vi "Flip FLop D (2).vi"() -> ()   [LabVIEW 2018]
panel:
  out "Q0*":bool
  in  "D0":bool
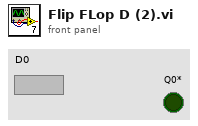
[diagram p1: front panel]
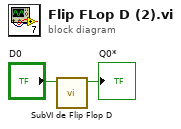
[diagram p0: block diagram]
diagram:
  n1 = call "SubVI de Flip Flop D.vi"("D0"="D0") -> ("Q0*"=→"Q0*":bool)  [unwired: 10 in]
